vi "lab session 8.1.vi"() -> ()   [LabVIEW 2020]
uses:
  <vilib>/numeric/Random Number (Range) U64.vi
  <vilib>/numeric/sub_Random U32.vi
panel:
  out "Waveform Chart":u64(graph)
  in  "stop":bool
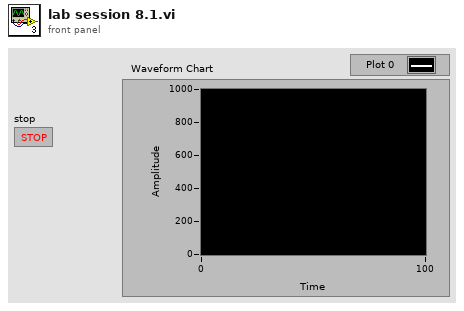
[diagram p1: front panel]
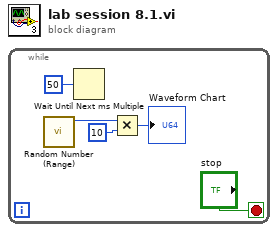
[diagram p0: block diagram]
diagram:
  n1 = while {
    stop <- "stop" stop-if-true
    n2 = call-poly <vilib>:"Random Number (Range).vi"() -> ("number"=w5:u64)  [unwired: 11 in]
    n3 = Wait Until Next ms Multiple(millisecond multiple=50) -> ()  [unwired: 1 out]
    n4 = Multiply(x=w5, y=u64 10) -> (x*y=→"Waveform Chart":u64)
  }
